vi "Benchmark 800kB Input.vi"() -> ()   [LabVIEW 2019]
uses:
  Base64_CharSet.vi
  Base64_ByteLUT.vi
  OpenSerializer.base64.lvlib
panel:
  out "bytes":i32
  out "Waveform Chart":cluster{dbl, dbl}(graph)
  out "OK":bool
  out "Encode":dbl
  out "Decode":dbl
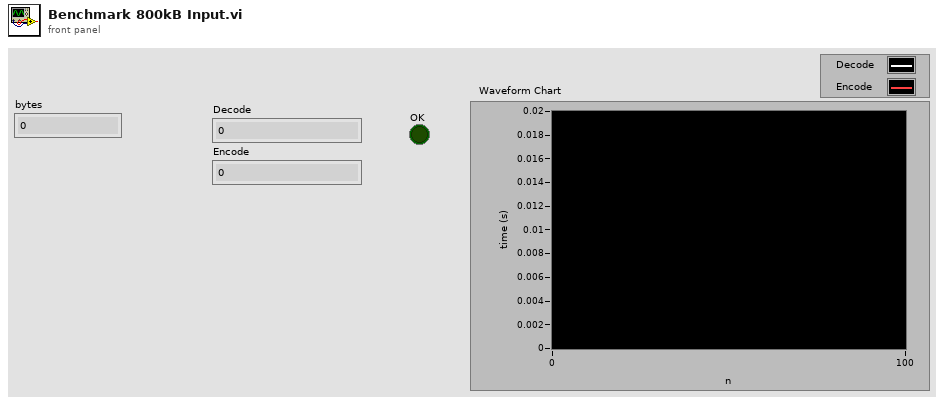
[diagram p1: front panel]
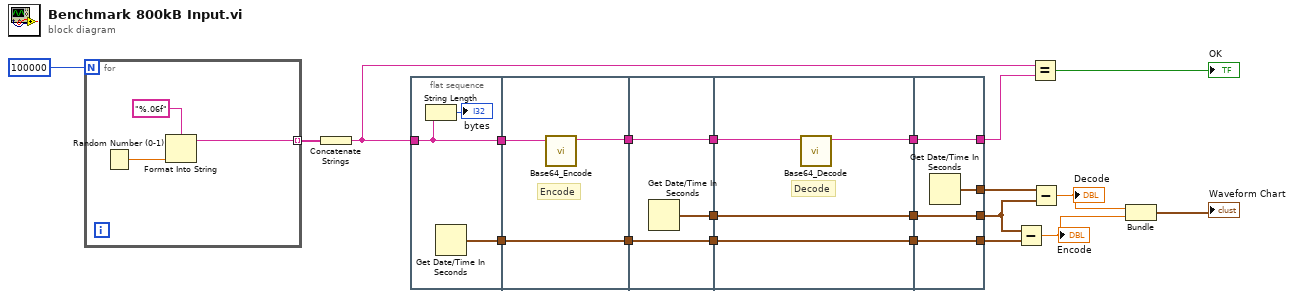
[diagram p0: block diagram]
diagram:
  n1 = for {
    N: 100000 ("Length x 8chars") -> [_]
    tunnel: [w23] -> w20 mode=indexing
    n2 = Random Number (0-1)() -> (number: 0 to 1=w24:dbl)
    n3 = Format Into String(format string="%.06f", w24) -> (resulting string=w23:string)  [unwired: 2 in, 1 out]
  }
  n4 = Concatenate Strings(w20) -> (w19:string)
  n5 = flat-sequence {
    tunnel: w19 -> [w26]
    tunnel: [w26] -> w18
    tunnel: [w27] -> w15
    tunnel: w18 -> [w29]
    tunnel: [w30] -> w17
    tunnel: [w28] -> w16
    tunnel: w15 -> [w28]
    tunnel: w17 -> [w31]
    tunnel: w16 -> [w32]
    tunnel: [w33] -> w14
    tunnel: [w32] -> w13
    tunnel: [w31] -> w1
    tunnel: w14 -> [w37]
    tunnel: w13 -> [w36]
    tunnel: [w37] -> w11
    tunnel: [w36] -> w10
    tunnel: [w35] -> w9
    tunnel: w1 -> [w34]
    tunnel: [w39] -> w12
    tunnel: [w40] -> w6
    tunnel: [w41] -> w7
    tunnel: w11 -> [w41]
    tunnel: w10 -> [w40]
    tunnel: w9 -> [w39]
    tunnel: [w38] -> w8
    frame #0 {
      n6 = String Length(string=w26) -> (length=→"bytes":i32)
      n7 = Get Date/Time In Seconds() -> (seconds since 1Jan1904=w27:timestamp)
    }
    frame #1 {
      # "Encode"
      n8 = call "Base64_Encode.vi"("String"=w29) -> ("Encoded String"=w30:string)  [unwired: 9 in, 1 out]
    }
    frame #2 {
      n9 = Get Date/Time In Seconds() -> (seconds since 1Jan1904=w33:timestamp)
    }
    frame #3 {
      # "Decode"
      n10 = call "Base64_Decode.vi"("Base64 String"=w34) -> ("Decoded String"=w35:string)  [unwired: 9 in, 1 out]
    }
    frame #4 {
      n11 = Get Date/Time In Seconds() -> (seconds since 1Jan1904=w38:timestamp)
    }
  }
  n12 = Subtract(x=w7, y=w6) -> (x-y=w3:dbl)
  "Encode" <- w3
  n13 = Equal?(x=w19, y=w12) -> (x = y?=→"OK":bool)
  n14 = Subtract(x=w8, y=w7) -> (x-y=w4:dbl)
  "Decode" <- w4
  n15 = Bundle(w4, w3) -> (→"Waveform Chart":cluster{dbl, dbl})  [unwired: 1 in]
